vi "Adjust Scroll.vi"(7 "Scroll Value":i32, 11 "Panels":refnum<class "Panel.lvclass">[](array[class])) -> (2 "Top Index":i32, 3 "DocMax":dbl, 5 "Fixed Value":i32)   [LabVIEW 2018]
uses:
  Panel/Panel.lvclass
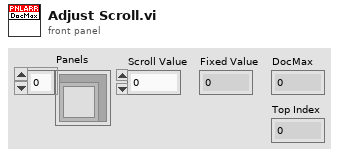
[diagram p1: front panel]
types:
  T1 = typedef "HalPanel.lvlib/Panel.lvclass/Desired Size.ctl" = cluster{"Width":i16, "Height":i16}
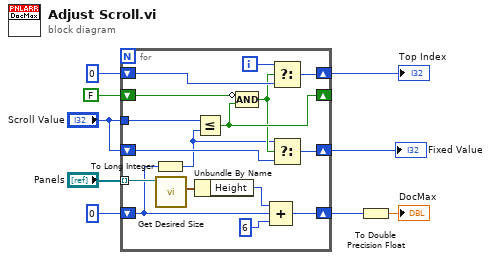
[diagram p0: block diagram]
diagram:
  n1 = for {
    tunnel: "Panels" -> [w25] mode=indexing
    shift-right: [w21] -> w7
    shift-left: i16 0 -> [w16]
    tunnel: "Scroll Value" -> [w18]
    shift-right: [w19] -> w4
    shift-left: 0 -> [w17]
    shift-right: [w14] -> _
    shift-left: FALSE -> [w15]
    shift-right: [w13] -> w1
    shift-left: "Scroll Value" -> [w12]
    i -> [w20]
    n2 = To Long Integer(number=w16) -> (32bit integer=w10:i32)
    n3 = call-dynamic "Get Desired Size.vi"("Panel in"=w25) -> ("Desired Size"=w24:T1)  [unwired: 8 in, 2 out]
    n4 = Less Or Equal?(x=w18, y=w10) -> (x <= y?=w14:bool)
    n5 = Unbundle By Name(w24) -> ("Height"=w22:i16)
    n6 = Compound Arithmetic op=AND(invert w15, w14) -> (w11:bool)
    n7 = Compound Arithmetic op=ADD(w22, w16, i16 6) -> (w21:i16)
    n8 = Select(t=w20, s=w11, f=w17) -> (s? t:f=w19:i32)
    n9 = Select(t=w10, s=w11, f=w12) -> (s? t:f=w13:i32)
  }
  "Top Index" <- w4
  "Fixed Value" <- w1
  n10 = To Double Precision Float(number=w7) -> (double precision float=→"DocMax":dbl)
